vi "Init Events.vi"(8 "error in (no error)":errorcluster, 11 "Entity Editor in":refnum<class "Entity Editor.lvclass">) -> (0 "error out":errorcluster, 3 "Entity Editor out":refnum<class "Entity Editor.lvclass">)   [LabVIEW 2020, in "Conditum-Tools.lvlib" / "Entity Editor.lvclass"]
uses:
  Entity Editor.lvclass
  Entity Editor.lvclass/Entity Editor.ctl
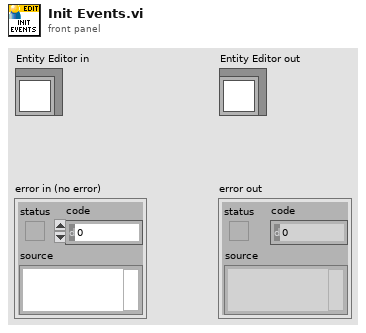
[diagram p1: front panel]
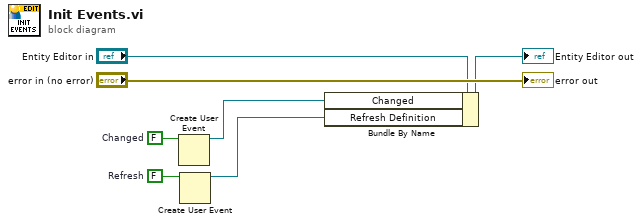
[diagram p0: block diagram]
diagram:
  w2 = FALSE  # Refresh
  w5 = FALSE  # Changed
  n1 = Create User Event(user event datatype=w5) -> (user event=w3:refnum<user-event>)  [unwired: 1 in, 1 out]
  n2 = Create User Event(user event datatype=w2) -> (user event=w1:refnum<user-event>)  [unwired: 1 in, 1 out]
  n3 = Bundle By Name(cluster="Entity Editor in", "Changed"=w3, "Refresh Definition"=w1) -> (→"Entity Editor out":refnum<class "Entity Editor.lvclass">)
  "error out" <- "error in (no error)"
